vi "Ist zu Grenzwert.vi"() -> (0 "maxLoop":i32, 3 "Grenzwerte Ist":T1={"Filter:"={"Sollwert"=0.0, "Warn-Min"=0.0, "Warn-Max"=0.0, "Abschalt-Min"=0.0, "Abschalt-Max"=0.0, "Regler"=1, "AnlagenParameter"=""}, "Ventilplatte:"={"Sollwert"=0.0, "Warn-Min"=0.0, "Warn-Max"=0.0, "Abschalt-Min"=0.0, "Abschalt-Max"=0.0, "Regler"=1, "AnlagenParameter"=""}, "Heizleitung 1:"={"Sollwert"=0.0, "Warn-Min"=0.0, "Warn-Max"=0.0, "Abschalt-Min"=0.0, "Abschalt-Max"=0.0, "Regler"=1, "AnlagenParameter"=""}, "Heizleitung 2:"={"Sollwert"=0.0, "Warn-Min"=0.0, "Warn-Max"=0.0, "Abschalt-Min"=0.0, "Abschalt-Max"=0.0, "Regler"=1, "AnlagenParameter"=""}, "Heizleitung 3:"={"Sollwert"=0.0, "Warn-Min"=0.0, "Warn-Max"=0.0, "Abschalt-Min"=0.0, "Abschalt-Max"=0.0, "Regler"=1, "AnlagenParameter"=""}, "Heizleitung 4:"={"Sollwert"=0.0, "Warn-Min"=0.0, "Warn-Max"=0.0, "Abschalt-Min"=0.0, "Abschalt-Max"=0.0, "Regler"=1, "AnlagenParameter"=""}, "Heizleitung 5:"={"Sollwert"=0.0, "Warn-Min"=0.0, "Warn-Max"=0.0, "Abschalt-Min"=0.0, "Abschalt-Max"=0.0, "Regler"=1, "AnlagenParameter"=""}, "Heizleitung 6:"={"Sollwert"=0.0, "Warn-Min"=0.0, "Warn-Max"=0.0, "Abschalt-Min"=0.0, "Abschalt-Max"=0.0, "Regler"=1, "AnlagenParameter"=""}} {"Heizleitung 6:"."Regler" items=["aktiv", "inaktiv"]; "Heizleitung 6:"."Abschalt-Max" format="%#_5g"; "Heizleitung 6:"."Abschalt-Min" format="%#_5g"; "Heizleitung 6:"."Warn-Max" format="%#_5g"; "Heizleitung 6:"."Warn-Min" format="%#_5g"; "Heizleitung 6:"."Sollwert" format="%#_5g"; "Heizleitung 5:"."Regler" items=["aktiv", "inaktiv"]; "Heizleitung 5:"."Abschalt-Max" format="%#_5g"; "Heizleitung 5:"."Abschalt-Min" format="%#_5g"; "Heizleitung 5:"."Warn-Max" format="%#_5g"; "Heizleitung 5:"."Warn-Min" format="%#_5g"; "Heizleitung 5:"."Sollwert" format="%#_5g"; "Heizleitung 4:"."Regler" items=["aktiv", "inaktiv"]; "Heizleitung 4:"."Abschalt-Max" format="%#_5g"; "Heizleitung 4:"."Abschalt-Min" format="%#_5g"; "Heizleitung 4:"."Warn-Max" format="%#_5g"; "Heizleitung 4:"."Warn-Min" format="%#_5g"; "Heizleitung 4:"."Sollwert" format="%#_5g"; "Heizleitung 3:"."Regler" items=["aktiv", "inaktiv"]; "Heizleitung 3:"."Abschalt-Max" format="%#_5g"; "Heizleitung 3:"."Abschalt-Min" format="%#_5g"; "Heizleitung 3:"."Warn-Max" format="%#_5g"; "Heizleitung 3:"."Warn-Min" format="%#_5g"; "Heizleitung 3:"."Sollwert" format="%#_5g"; "Heizleitung 2:"."Regler" items=["aktiv", "inaktiv"]; "Heizleitung 2:"."Abschalt-Max" format="%#_5g"; "Heizleitung 2:"."Abschalt-Min" format="%#_5g"; "Heizleitung 2:"."Warn-Max" format="%#_5g"; "Heizleitung 2:"."Warn-Min" format="%#_5g"; "Heizleitung 2:"."Sollwert" format="%#_5g"; "Heizleitung 1:"."Regler" items=["aktiv", "inaktiv"]; "Heizleitung 1:"."Abschalt-Max" format="%#_5g"; "Heizleitung 1:"."Abschalt-Min" format="%#_5g"; "Heizleitung 1:"."Warn-Max" format="%#_5g"; "Heizleitung 1:"."Warn-Min" format="%#_5g"; "Heizleitung 1:"."Sollwert" format="%#_5g"; "Ventilplatte:"."Regler" items=["aktiv", "inaktiv"]; "Ventilplatte:"."Abschalt-Max" format="%#_5g"; "Ventilplatte:"."Abschalt-Min" format="%#_5g"; "Ventilplatte:"."Warn-Max" format="%#_5g"; "Ventilplatte:"."Warn-Min" format="%#_5g"; "Ventilplatte:"."Sollwert" format="%#_5g"; "Filter:"."Regler" items=["aktiv", "inaktiv"]; "Filter:"."Abschalt-Max" format="%#_5g"; "Filter:"."Abschalt-Min" format="%#_5g"; "Filter:"."Warn-Max" format="%#_5g"; "Filter:"."Warn-Min" format="%#_5g"; "Filter:"."Sollwert" format="%#_5g"})   [LabVIEW 2020, in "PNS.lvlib"]
uses:
  PNS.lvlib
  ObjektKlassen/Steuerung PNS/Anlegengrenzwerte PNS.ctl
  ObjektKlassen/Steuerung PNS/Anlagengrenzwerte Parameteranzeige.ctl
  Visualisierungs Elemente/Zahlen-Eingabefeld.ctl
  Aktionen FGV Istwerte.ctl
  Aktionen FGV Loopkennung.ctl
  ObjektKlassen/Steuerung PNS/Steuerung PNS.lvclass
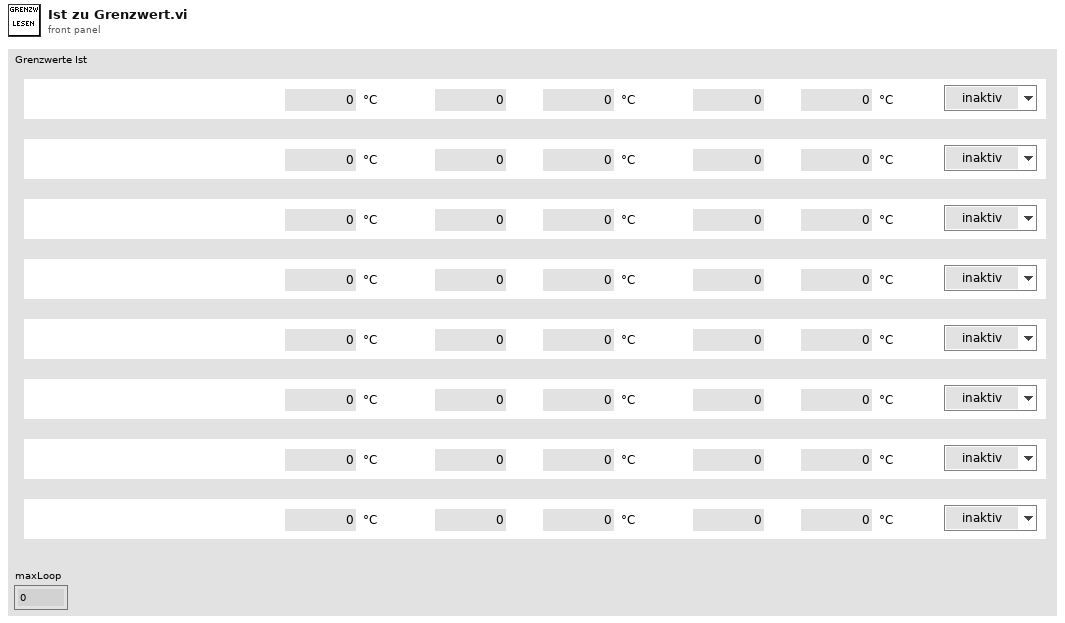
[diagram p1: front panel]
types:
  T1 = typedef "Steuerung PNS.lvclass/Anlegengrenzwerte PNS.ctl" = cluster{"Filter:":T2, "Ventilplatte:":T2, "Heizleitung 1:":T2, "Heizleitung 2:":T2, "Heizleitung 3:":T2, "Heizleitung 4:":T2, "Heizleitung 5:":T2, "Heizleitung 6:":T2}
  T2 = typedef "Steuerung PNS.lvclass/Anlagengrenzwerte Parameteranzeige.ctl" = cluster{"Sollwert":T3, "Warn-Min":T3, "Warn-Max":T3, "Abschalt-Min":T3, "Abschalt-Max":T3, "Regler":u16, "AnlagenParameter":string}
  T3 = typedef "Zahlen-Eingabefeld.ctl" = sgl
  T4 = typedef "PNS.lvlib/Aktionen FGV Loopkennung.ctl" = enum16{"lesen", "schreiben"}
  T5 = typedef "PNS.lvlib/Aktionen FGV Istwerte.ctl" = enum16{"lesen", "initialisieren", "schreiben", "Störungen"}
  T6 = typedef "Steuerung PNS.lvclass/Regler.ctl" = cluster{"Istwert":i16, "Sollwert":i16, "Alarm MIN":i16, "Alarm MAX":i16, "Regler sperren":i16, "Analog Ausgang":i16}[]
  T7 = typedef "Steuerung PNS.lvclass/Alarme.ctl" = cluster{"Alarm Filter max":u16, "Alarm Filter min":u16, "Alarm Ventilplatte max":u16, "Alarm Ventilplatte min":u16, "Alarm HL1 max":u16, "Alarm HL1 min":u16, "Alarm HL2 max":u16, "Alarm HL2 min":u16, "Alarm HL3 max":u16, "Alarm HL3 min":u16, "Alarm HL4 max":u16, "Alarm HL4 min":u16, "Alarm HL5 max":u16, "Alarm HL5 min":u16, "Alarm HL6 max":u16, "Alarm HL6 min":u16}
  T8 = cluster{"Loops":string[], "Gerätetype":string, "Loopkennung":u16[], "Seriennummer":string, "Geraetekennung":u16, "SoftWare Version":string}
  T9 = cluster{"Istwert":i16, "Sollwert":i16, "Alarm MIN":i16, "Alarm MAX":i16, "Regler sperren":i16, "Analog Ausgang":i16}
  T10 = cluster{"Sollwert":i16, "Alarm Filter min":u16, "Alarm Filter max":u16, "Alarm Filter min":u16, "Alarm Filter max":u16, "Regler sperren":i16, string}
  T11 = cluster{"Sollwert":i16, "Alarm Ventilplatte min":u16, "Alarm Ventilplatte max":u16, "Alarm Ventilplatte min":u16, "Alarm Ventilplatte max":u16, "Regler sperren":i16, string}
  T12 = cluster{"Sollwert":i16, "Alarm HL1 min":u16, "Alarm HL1 max":u16, "Alarm HL1 min":u16, "Alarm HL1 max":u16, "Regler sperren":i16, string}
  T13 = cluster{"Sollwert":i16, "Alarm HL2 min":u16, "Alarm HL2 max":u16, "Alarm HL2 min":u16, "Alarm HL2 max":u16, "Regler sperren":i16, string}
  T14 = cluster{"Sollwert":i16, "Alarm HL3 min":u16, "Alarm HL3 max":u16, "Alarm HL3 min":u16, "Alarm HL3 max":u16, "Regler sperren":i16, string}
  T15 = cluster{"Sollwert":i16, "Alarm HL4 min":u16, "Alarm HL4 max":u16, "Alarm HL4 min":u16, "Alarm HL4 max":u16, "Regler sperren":i16, string}
  T16 = cluster{"Sollwert":i16, "Alarm HL5 min":u16, "Alarm HL5 max":u16, "Alarm HL5 min":u16, "Alarm HL5 max":u16, "Regler sperren":i16, string}
  T17 = cluster{"Sollwert":i16, "Alarm HL6 min":u16, "Alarm HL6 max":u16, "Alarm HL6 min":u16, "Alarm HL6 max":u16, "Regler sperren":i16, string}
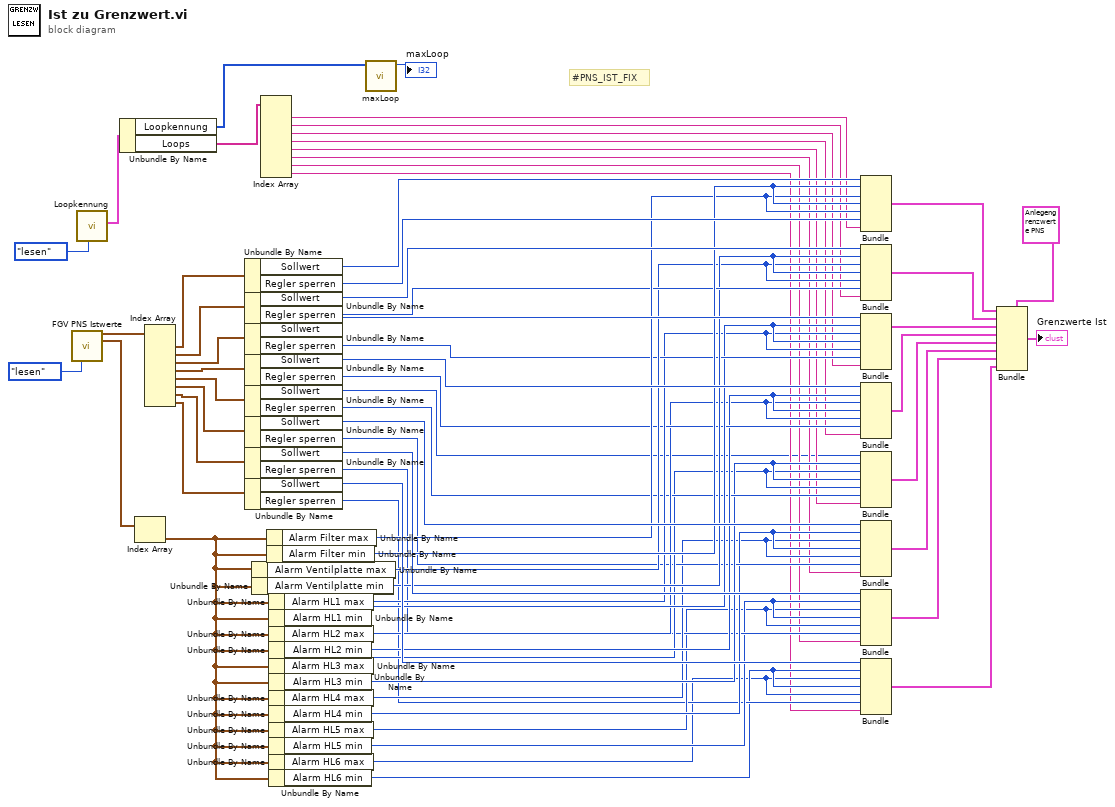
[diagram p0: block diagram]
diagram:
  # "#PNS_IST_FIX"
  n1 = call "FGV PNS Istwerte.vi"("Aktionen"=Aktionen_FGV_Istwerte."lesen") -> ("Regler"=w7:T6, "Alarme"=w6:T7[])  [unwired: 11 in, 2 out]
  n2 = call "Loopkennung.vi"("Aktion"=Aktionen_FGV_Loopkennung."lesen") -> ("LoopGeraetekennung"=w5:T8)  [unwired: 9 in, 1 out]
  n3 = Unbundle By Name(w5) -> ("Loopkennung"=w2:u16[], "Loops"=w17:string[])
  n4 = Index Array(array=w6) -> (element=w42:T7)  [unwired: 1 in]
  n5 = Index Array(array=w7) -> (element #1=w44:T9, element #2=w45:T9, element #3=w46:T9, element #4=w47:T9, element #5=w48:T9, element #6=w49:T9, element #7=w50:T9, element #8=w51:T9)  [unwired: 8 in]
  n6 = Unbundle By Name(w44) -> ("Sollwert"=w52:i16, "Regler sperren"=w41:i16)
  n7 = Unbundle By Name(w45) -> ("Sollwert"=w54:i16, "Regler sperren"=w38:i16)
  n8 = Unbundle By Name(w46) -> ("Sollwert"=w43:i16, "Regler sperren"=w35:i16)
  n9 = Unbundle By Name(w47) -> ("Sollwert"=w62:i16, "Regler sperren"=w32:i16)
  n10 = Unbundle By Name(w48) -> ("Sollwert"=w8:i16, "Regler sperren"=w29:i16)
  n11 = Unbundle By Name(w49) -> ("Sollwert"=w63:i16, "Regler sperren"=w26:i16)
  n12 = Unbundle By Name(w50) -> ("Sollwert"=w64:i16, "Regler sperren"=w23:i16)
  n13 = Unbundle By Name(w51) -> ("Sollwert"=w65:i16, "Regler sperren"=w20:i16)
  n14 = Unbundle By Name(w42) -> ("Alarm Ventilplatte max"=w36:u16)
  n15 = Unbundle By Name(w42) -> ("Alarm Ventilplatte min"=w37:u16)
  n16 = Index Array(array=w17) -> (element #1=w16:string, element #2=w15:string, element #3=w14:string, element #4=w13:string, element #5=w12:string, element #6=w11:string, element #7=w10:string, element #8=w9:string)  [unwired: 8 in]
  n17 = Unbundle By Name(w42) -> ("Alarm Filter max"=w39:u16)
  n18 = Unbundle By Name(w42) -> ("Alarm Filter min"=w40:u16)
  n19 = Unbundle By Name(w42) -> ("Alarm HL1 max"=w33:u16)
  n20 = Unbundle By Name(w42) -> ("Alarm HL1 min"=w34:u16)
  n21 = Unbundle By Name(w42) -> ("Alarm HL2 max"=w30:u16)
  n22 = Unbundle By Name(w42) -> ("Alarm HL2 min"=w31:u16)
  n23 = Unbundle By Name(w42) -> ("Alarm HL3 max"=w27:u16)
  n24 = Unbundle By Name(w42) -> ("Alarm HL3 min"=w28:u16)
  n25 = Unbundle By Name(w42) -> ("Alarm HL4 max"=w24:u16)
  n26 = Unbundle By Name(w42) -> ("Alarm HL4 min"=w25:u16)
  n27 = Unbundle By Name(w42) -> ("Alarm HL5 max"=w21:u16)
  n28 = Unbundle By Name(w42) -> ("Alarm HL5 min"=w22:u16)
  n29 = Unbundle By Name(w42) -> ("Alarm HL6 max"=w18:u16)
  n30 = Unbundle By Name(w42) -> ("Alarm HL6 min"=w19:u16)
  n31 = call "maxLoop.vi"("Loopkennung"=w2) -> ("Numerisch"=→"maxLoop":i32)  [unwired: 10 in]
  n32 = Bundle("Sollwert"=w52, "Alarm Filter min"=w40, "Alarm Filter max"=w39, "Alarm Filter min"=w40, "Alarm Filter max"=w39, "Regler sperren"=w41, w16) -> (w53:T10)  [unwired: 1 in]
  n33 = Bundle("Sollwert"=w54, "Alarm Ventilplatte min"=w37, "Alarm Ventilplatte max"=w36, "Alarm Ventilplatte min"=w37, "Alarm Ventilplatte max"=w36, "Regler sperren"=w38, w15) -> (w55:T11)  [unwired: 1 in]
  n34 = Bundle("Sollwert"=w43, "Alarm HL1 min"=w34, "Alarm HL1 max"=w33, "Alarm HL1 min"=w34, "Alarm HL1 max"=w33, "Regler sperren"=w35, w14) -> (w56:T12)  [unwired: 1 in]
  n35 = Bundle("Sollwert"=w62, "Alarm HL2 min"=w31, "Alarm HL2 max"=w30, "Alarm HL2 min"=w31, "Alarm HL2 max"=w30, "Regler sperren"=w32, w13) -> (w57:T13)  [unwired: 1 in]
  n36 = Bundle("Sollwert"=w8, "Alarm HL3 min"=w28, "Alarm HL3 max"=w27, "Alarm HL3 min"=w28, "Alarm HL3 max"=w27, "Regler sperren"=w29, w12) -> (w58:T14)  [unwired: 1 in]
  n37 = Bundle("Sollwert"=w63, "Alarm HL4 min"=w25, "Alarm HL4 max"=w24, "Alarm HL4 min"=w25, "Alarm HL4 max"=w24, "Regler sperren"=w26, w11) -> (w59:T15)  [unwired: 1 in]
  n38 = Bundle("Sollwert"=w64, "Alarm HL5 min"=w22, "Alarm HL5 max"=w21, "Alarm HL5 min"=w22, "Alarm HL5 max"=w21, "Regler sperren"=w23, w10) -> (w60:T16)  [unwired: 1 in]
  n39 = Bundle("Sollwert"=w65, "Alarm HL6 min"=w19, "Alarm HL6 max"=w18, "Alarm HL6 min"=w19, "Alarm HL6 max"=w18, "Regler sperren"=w20, w9) -> (w61:T17)  [unwired: 1 in]
  n40 = Bundle(cluster=T1 {"Filter:"={"Sollwert"=0.0, "Warn-Min"=0.0, "Warn-Max"=0.0, "Abschalt-Min"=0.0, "Abschalt-Max"=0.0, "Regler"=1, "AnlagenParameter"=""}, "Ventilplatte:"={"Sollwert"=0.0, "Warn-Min"=0.0, "Warn-Max"=0.0, "Abschalt-Min"=0.0, "Abschalt-Max"=0.0, "Regler"=1, "AnlagenParameter"=""}, "Heizleitung 1:"={"Sollwert"=0.0, "Warn-Min"=0.0, "Warn-Max"=0.0, "Abschalt-Min"=0.0, "Abschalt-Max"=0.0, "Regler"=1, "AnlagenParameter"=""}, "Heizleitung 2:"={"Sollwert"=0.0, "Warn-Min"=0.0, "Warn-Max"=0.0, "Abschalt-Min"=0.0, "Abschalt-Max"=0.0, "Regler"=1, "AnlagenParameter"=""}, "Heizleitung 3:"={"Sollwert"=0.0, "Warn-Min"=0.0, "Warn-Max"=0.0, "Abschalt-Min"=0.0, "Abschalt-Max"=0.0, "Regler"=1, "AnlagenParameter"=""}, "Heizleitung 4:"={"Sollwert"=0.0, "Warn-Min"=0.0, "Warn-Max"=0.0, "Abschalt-Min"=0.0, "Abschalt-Max"=0.0, "Regler"=1, "AnlagenParameter"=""}, "Heizleitung 5:"={"Sollwert"=0.0, "Warn-Min"=0.0, "Warn-Max"=0.0, "Abschalt-Min"=0.0, "Abschalt-Max"=0.0, "Regler"=1, "AnlagenParameter"=""}, "Heizleitung 6:"={"Sollwert"=0.0, "Warn-Min"=0.0, "Warn-Max"=0.0, "Abschalt-Min"=0.0, "Abschalt-Max"=0.0, "Regler"=1, "AnlagenParameter"=""}} ("Grenzwerte PNS"), "Filter:"=w53, "Ventilplatte:"=w55, "Heizleitung 1:"=w56, "Heizleitung 2:"=w57, "Heizleitung 3:"=w58, "Heizleitung 4:"=w59, "Heizleitung 5:"=w60, "Heizleitung 6:"=w61) -> (→"Grenzwerte Ist":T1)
